vi "DSF.Engine.Status.Framework.Create.vi"(8 "error in (no error)":errorcluster) -> (0 "error out":errorcluster, 3 "Framework Status":refnum<class "DSF.Engine.Status.Framework.lvclass">)   [LabVIEW 2017, in "Data Sharing Framework Engine.lvlib" / "DSF.Engine.Status.Framework.lvclass"]
uses:
  DSF.Engine.Status.Framework.lvclass
  DSF.Engine.Status.Framework.lvclass/DSF.Engine.Status.Framework.ctl
  DSF.Engine.Status.Framework.Performance.lvclass
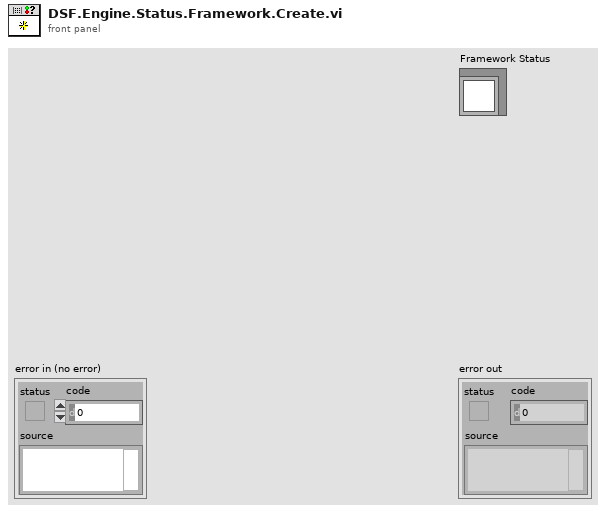
[diagram p1: front panel]
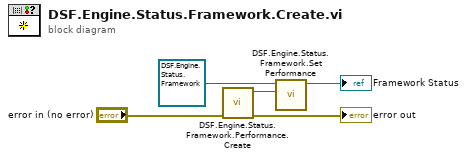
[diagram p0: block diagram]
diagram:
  n1 = call "DSF.Engine.Status.Framework.Performance.Create.vi"("error in (no error)"="error in (no error)") -> ("error out"=→"error out":errorcluster, "Framework Performance"=w3:refnum<class "DSF.Engine.Status.Framework.Performance.lvclass">)  [unwired: 9 in]
  n2 = call "DSF.Engine.Status.Framework.Set Performance.vi"("Framework Performance"=w3, "Framework Status in"=refnum<class "DSF.Engine.Status.Framework.lvclass"> refnum) -> ("Framework Status out"=→"Framework Status":refnum<class "DSF.Engine.Status.Framework.lvclass">)  [unwired: 9 in]
